vi "2 PulseGenerations.vi"(2 "PulseGen Packets":u64[](array[numeric])=[0, 0], 4 "2 PulseGen Chs":cluster{"DO0":refnum<k21>, "DO1":refnum<k21>}={"DO0"="Connector0/DIO4", "DO1"="Connector0/DIO5"}) -> ()   [LabVIEW 2010]
uses:
  <vilib>/eio/EIONode/EIONode.xnode
  <vilib>/rvi/eio/nirviEIOImplementation/nirviEIOImplementation.xnode
  <vilib>/rvi/eio/common/nirviEmuClasses.ctl
  <vilib>/rvi/eio/common/nirviEmuTemplateMethod_noerrors.vi
  <vilib>/NI Veristand/FPGA/NI_VS FPGA Support.lvlib
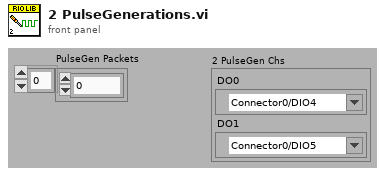
[diagram p1: front panel]
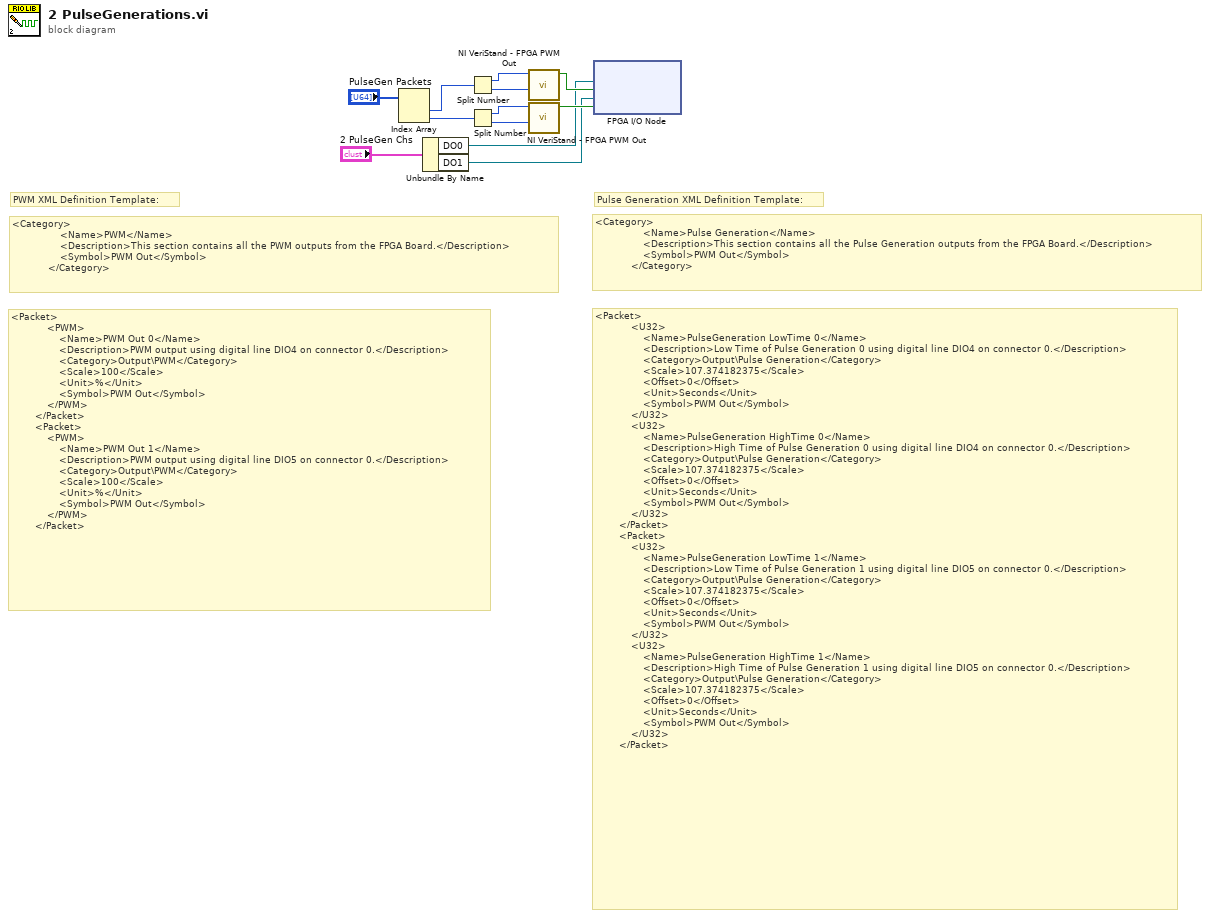
[diagram p0: block diagram]
diagram:
  # "<Category>\n                <Name>Pulse Generation</Name>\n                <Description>This section contains all the Pulse Generation outputs from the FPGA Board.</Description>\n                <Symbol>PWM Out</Symbol>\n            </Category>"
  # "<Category>\n                <Name>PWM</Name>\n                <Description>This section contains all the PWM outputs from the FPGA Board.</Description>\n                <Symbol>PWM Out</Symbol>\n            </Category>"
  # "<Packet>\n            <U32>\n                <Name>PulseGeneration LowTime 0</Name>\n                <Description>Low Time of Pulse Generation 0 using digital line DIO4 on connector 0.</Description>\n                <Category>Output\\Pulse Generation</Category>\n                <Scale>107.374182375</Scale>\n                <Offset>0</Offset>\n                <Unit>Seconds</Unit>\n                <Symbol>PWM Out</Symbol>\n            </U32>\n            <U32>\n                <Name>PulseGeneration HighTime 0</Name>\n                <Description>High Time of Pulse Generation 0 using digital line DIO4 on connector 0.</Description>\n                <Category>Output\\Pulse Generation</Category>\n                <Scale>107.374182375</Scale>\n                <Offset>0</Offset>\n                <Unit>Seconds</Unit>\n                <Symbol>PWM Out</Symbol>\n            </U32>\n        </Packet>\n        <Packet>\n            <U32>\n                <Name>PulseGeneration LowTime 1</Name>\n                <Description>Low Time of Pulse Generation 1 using digital line DIO5 on connector 0.</Description>\n                <Category>Output\\Pulse Generation</Category>\n                <Scale>107.374182375</Scale>\n                <Offset>0</Offset>\n                <Unit>Seconds</Unit>\n                <Symbol>PWM Out</Symbol>\n            </U32>\n            <U32>\n                <Name>PulseGeneration HighTime 1</Name>\n                <Description>High Time of Pulse Generation 1 using digital line DIO5 on connector 0.</Description>\n                <Category>Output\\Pulse Generation</Category>\n                <Scale>107.374182375</Scale>\n                <Offset>0</Offset>\n                <Unit>Seconds</Unit>\n                <Symbol>PWM Out</Symbol>\n            </U32>\n        </Packet>"
  # "<Packet>\n            <PWM>\n                <Name>PWM Out 0</Name>\n                <Description>PWM output using digital line DIO4 on connector 0.</Description>\n                <Category>Output\\PWM</Category>\n                <Scale>100</Scale>\n                <Unit>%</Unit>\n                <Symbol>PWM Out</Symbol>\n            </PWM>\n        </Packet>\n        <Packet>\n            <PWM>\n                <Name>PWM Out 1</Name>\n                <Description>PWM output using digital line DIO5 on connector 0.</Description>\n                <Category>Output\\PWM</Category>\n                <Scale>100</Scale>\n                <Unit>%</Unit>\n                <Symbol>PWM Out</Symbol>\n            </PWM>\n        </Packet>"
  # "Pulse Generation XML Definition Template:"
  # "PWM XML Definition Template:"
  n1 = Index Array(array="PulseGen Packets") -> (element #1=w10:u64, element #2=w11:u64)  [unwired: 2 in]
  n2 = Unbundle By Name("2 PulseGen Chs") -> ("DO0"=w2:refnum<k21>, "DO1"=w1:refnum<k21>)
  n3 = Split Number(x=w10) -> (hi(x)=w5:u32, lo(x)=w6:u32)
  n4 = Split Number(x=w11) -> (hi(x)=w8:u32, lo(x)=w7:u32)
  n5 = call <vilib>:"NI VeriStand - FPGA PWM Out.vi"("_Low Time"=w6, "_High Time"=w5) -> ("Output"=w4:bool)  [unwired: 1 in, 8 out]
  n6 = call <vilib>:"NI VeriStand - FPGA PWM Out.vi"("_Low Time"=w7, "_High Time"=w8) -> ("Output"=w12:bool)  [unwired: 1 in, 8 out]
  n7 = xnode "FPGA I/O Node"("I/O Item"=w4, "I/O Item"=w12, "FPGA I/O In"=w2, "FPGA I/O In"=w1) -> ()  [unwired: 2 out]
